vi "Test 3D String.vi"() -> ()   [LabVIEW 2014]
panel:
  out "String":string
  in  "Message":string="STATUS"
  in  "To":string="M"
  in  "From":string="A"
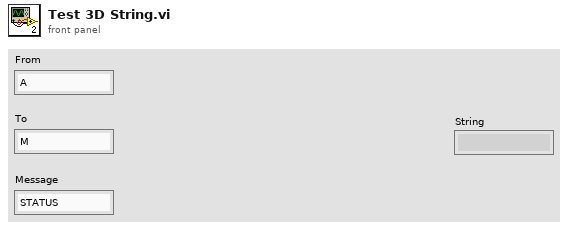
[diagram p1: front panel]
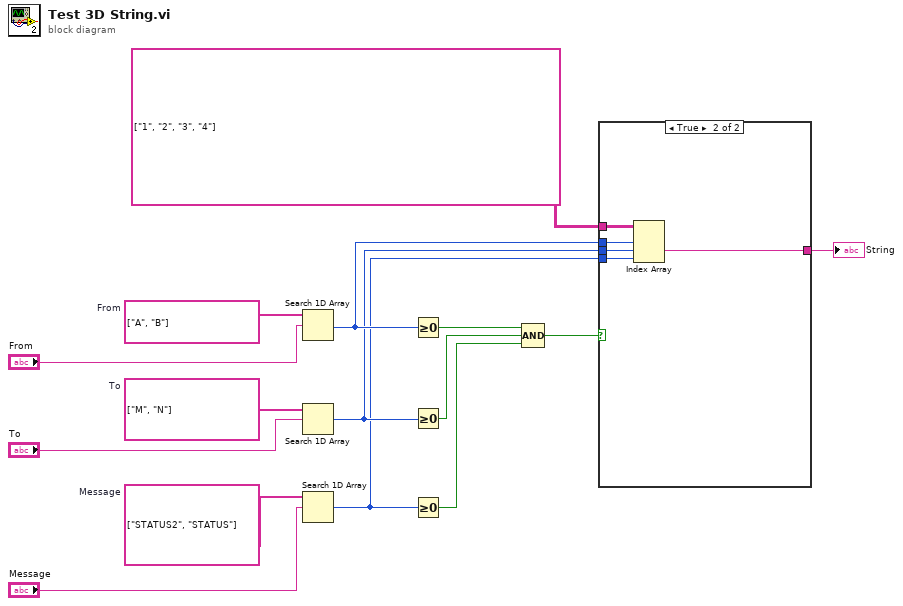
[diagram p0: block diagram]
diagram:
  w13 = string[] ["STATUS2", "STATUS"]  # Message
  w14 = string[] ["M", "N"]  # To
  w15 = string[] ["A", "B"]  # From
  n1 = Search 1D Array(1D array=w15, element="From") -> (index of element=w4:i32)  [unwired: 1 in]
  n2 = Search 1D Array(1D array=w14, element="To") -> (index of element=w3:i32)  [unwired: 1 in]
  n3 = Search 1D Array(1D array=w13, element="Message") -> (index of element=w2:i32)  [unwired: 1 in]
  n4 = Greater Or Equal To 0?(x=w4) -> (x >= 0?=w12:bool)
  n5 = Greater Or Equal To 0?(x=w3) -> (x >= 0?=w11:bool)
  n6 = Greater Or Equal To 0?(x=w2) -> (x >= 0?=w10:bool)
  n7 = Compound Arithmetic op=AND(w12, w11, w10) -> (w6:bool)
  n8 = case shown="True" w6 {
    tunnel: string[][][] [[["1", "2"], ["3", "4"]]] -> [_ w20]
    tunnel: w4 -> [_ w19]
    tunnel: w3 -> [_ w18]
    tunnel: w2 -> [_ w17]
    tunnel: [_ w16] -> w1
    frame False {
    }
    frame True {
      n9 = Index Array(array=w20, index (dim 0)=w19, index (dim 1)=w18, index (dim 2)=w17) -> (element=w16:string)
    }
  }
  "String" <- w1
